vi "twoMPU.vi"() -> ()   [LabVIEW 2016]
uses:
  <vilib>/MakerHub/LINX/Private/Type Defs/Interface.ctl
  <vilib>/MakerHub/LINX/Public/Sensors/Accelerometer/MPU60X0/Clock Source.ctl
  Control 1.ctl
  <vilib>/MakerHub/LINX/Private/Type Defs/User Platform.ctl
  <vilib>/MakerHub/LINX/Public/Sensors/Accelerometer/MPU60X0/DeviceAddresses.ctl
  <vilib>/MakerHub/LINX/Public/Sensors/Accelerometer/MPU60X0/AccelFullScaleRanges.ctl
  <vilib>/MakerHub/LINX/Public/Sensors/Accelerometer/MPU60X0/GyroFullScaleRanges.ctl
  <vilib>/MakerHub/LINX/Public/Initialize.vi
  <vilib>/MakerHub/LINX/LMH-LINX.lvlib
  <vilib>/MakerHub/LINX/Public/Sensors/Accelerometer/MPU60X0/MPU60X0.lvlib
  <vilib>/Platform/NI_3dgraph.lvlib
panel:
  in  "DATA RECORD":bool
  out "XY Graph 2":cluster{"Y":dbl[], "Y":dbl[]}[](graph)
  out "Path Length 2":dbl
  in  "Baud Rate Override":T1
  in  "Clock Source 2":T2
  out "Path Length":dbl
  out "vector error":errorcluster
  in  "Plot of roll and pitch":refnum<k7>(container)
  out "XY Graph":cluster{"Y":dbl[], "Y":dbl[]}[](graph)
  out "error out":errorcluster
  out "MATLAB Error":errorcluster
  out "Error Out":errorcluster
  in  "?":bool
  in  "I2C Channel":u8
  in  "Clock Source":T2
  in  "Interface":T3
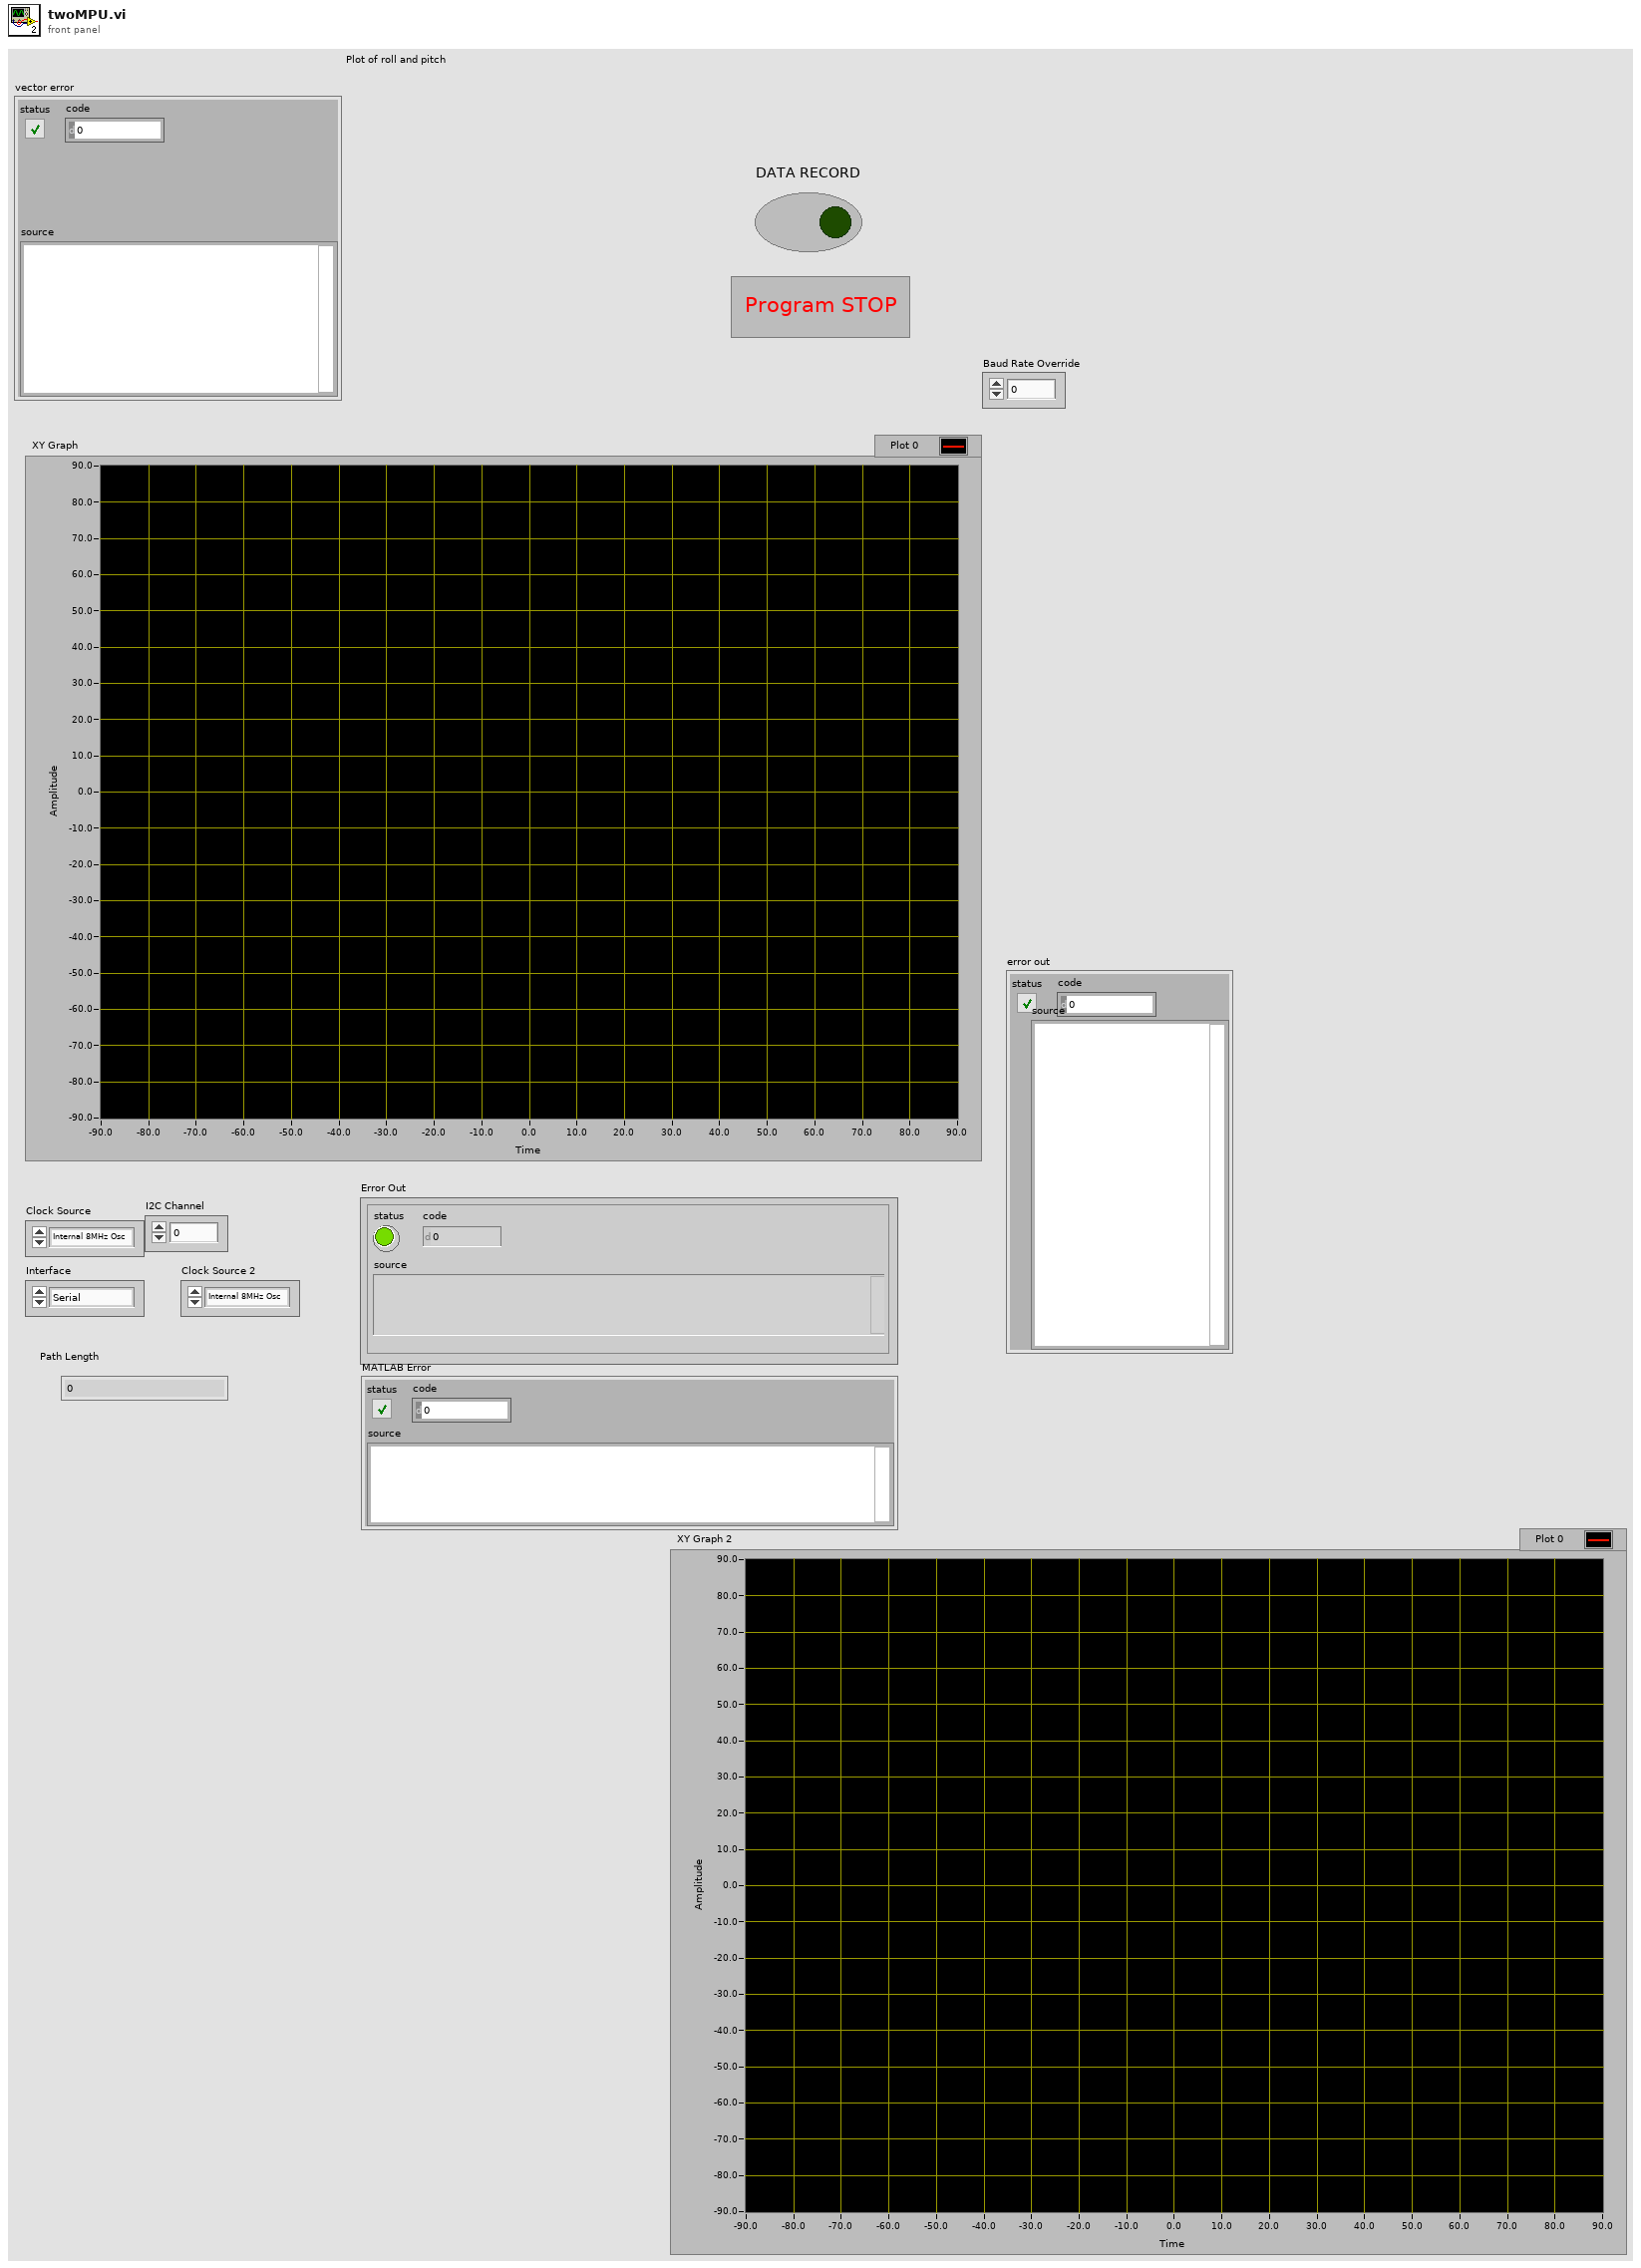
[diagram p1: front panel]
types:
  T1 = typedef "Control 1.ctl" = u32
  T2 = typedef "LMH-LINX.lvlib/MPU60X0.lvlib/Clock Source.ctl" = enum8{"Internal 8MHz Osc", "PLL with X Gyro Ref", "PLL with Y Gyro Ref", "PLL with Z Gyro Ref", "PLL with ext 32.768 KHz Ref", "PLL with ext 19.2 MHz Ref", "Reserved", "Hold in reset"}
  T3 = typedef "LMH-LINX.lvlib/Interface.ctl" = enum16{"Serial", "TCP"}
  T4 = typedef "LMH-LINX.lvlib/MPU60X0.lvlib/DeviceAddresses.ctl" = enum16{"0x68", "0x69"}
  T5 = typedef "LMH-LINX.lvlib/MPU60X0.lvlib/GyroFullScaleRanges.ctl" = enum8{"±250 °/s", "±500 °/s", "±1000 °/s", "±2000 °/s"}
  T6 = typedef "LMH-LINX.lvlib/MPU60X0.lvlib/AccelFullScaleRanges.ctl" = enum16{"±2g", "±4g", "±8g", "±16g"}
  T7 = typedef "LMH-LINX.lvlib/User Platform.ctl" = enum16{"Default", "Remote", "Local"}
  T8 = typedef "LMH-LINX.lvlib/LINX Ref.ctl" = cluster{"IO":T9, "Interface":T3, "LINX Device Config":T10}
  T9 = typedef "LMH-LINX.lvlib/Platform.ctl" = enum16{"Remote", "Local"}
  T10 = typedef "LMH-LINX.lvlib/Device.lvlib/LINX Device Config.ctl" = cluster{"Interface":T3, "COM Port":refnum<visa-resource-name>, "TCP Configuration":T11, "Device Family":u8, "Device ID":u8, "Device Name":string, "TCP Ref":refnum<k5>, "Channels":T12}
  T11 = typedef "LMH-LINX.lvlib/Device.lvlib/TCP Config.ctl" = cluster{"IP Address":string, "Port":u16}
  T12 = typedef "LMH-LINX.lvlib/Channels.ctl" = cluster{"DI":u8[], "DO":u8[], "AI":u8[], "AO":u8[], "PWM":u8[], "QE":u8[], "UART":u8[], "I2C 2":u8[], "SPI":u8[], "CAN":u8[], "Servo":u8[], "AI Ref (V)":dbl, "AI Resolution (Bits)":u8, "AO Ref (V)":dbl, "AO Resolution (Bits)":u8}
  T13 = cluster{"X Axis":i16, "Y Axis":i16, "Z Axis":i16}
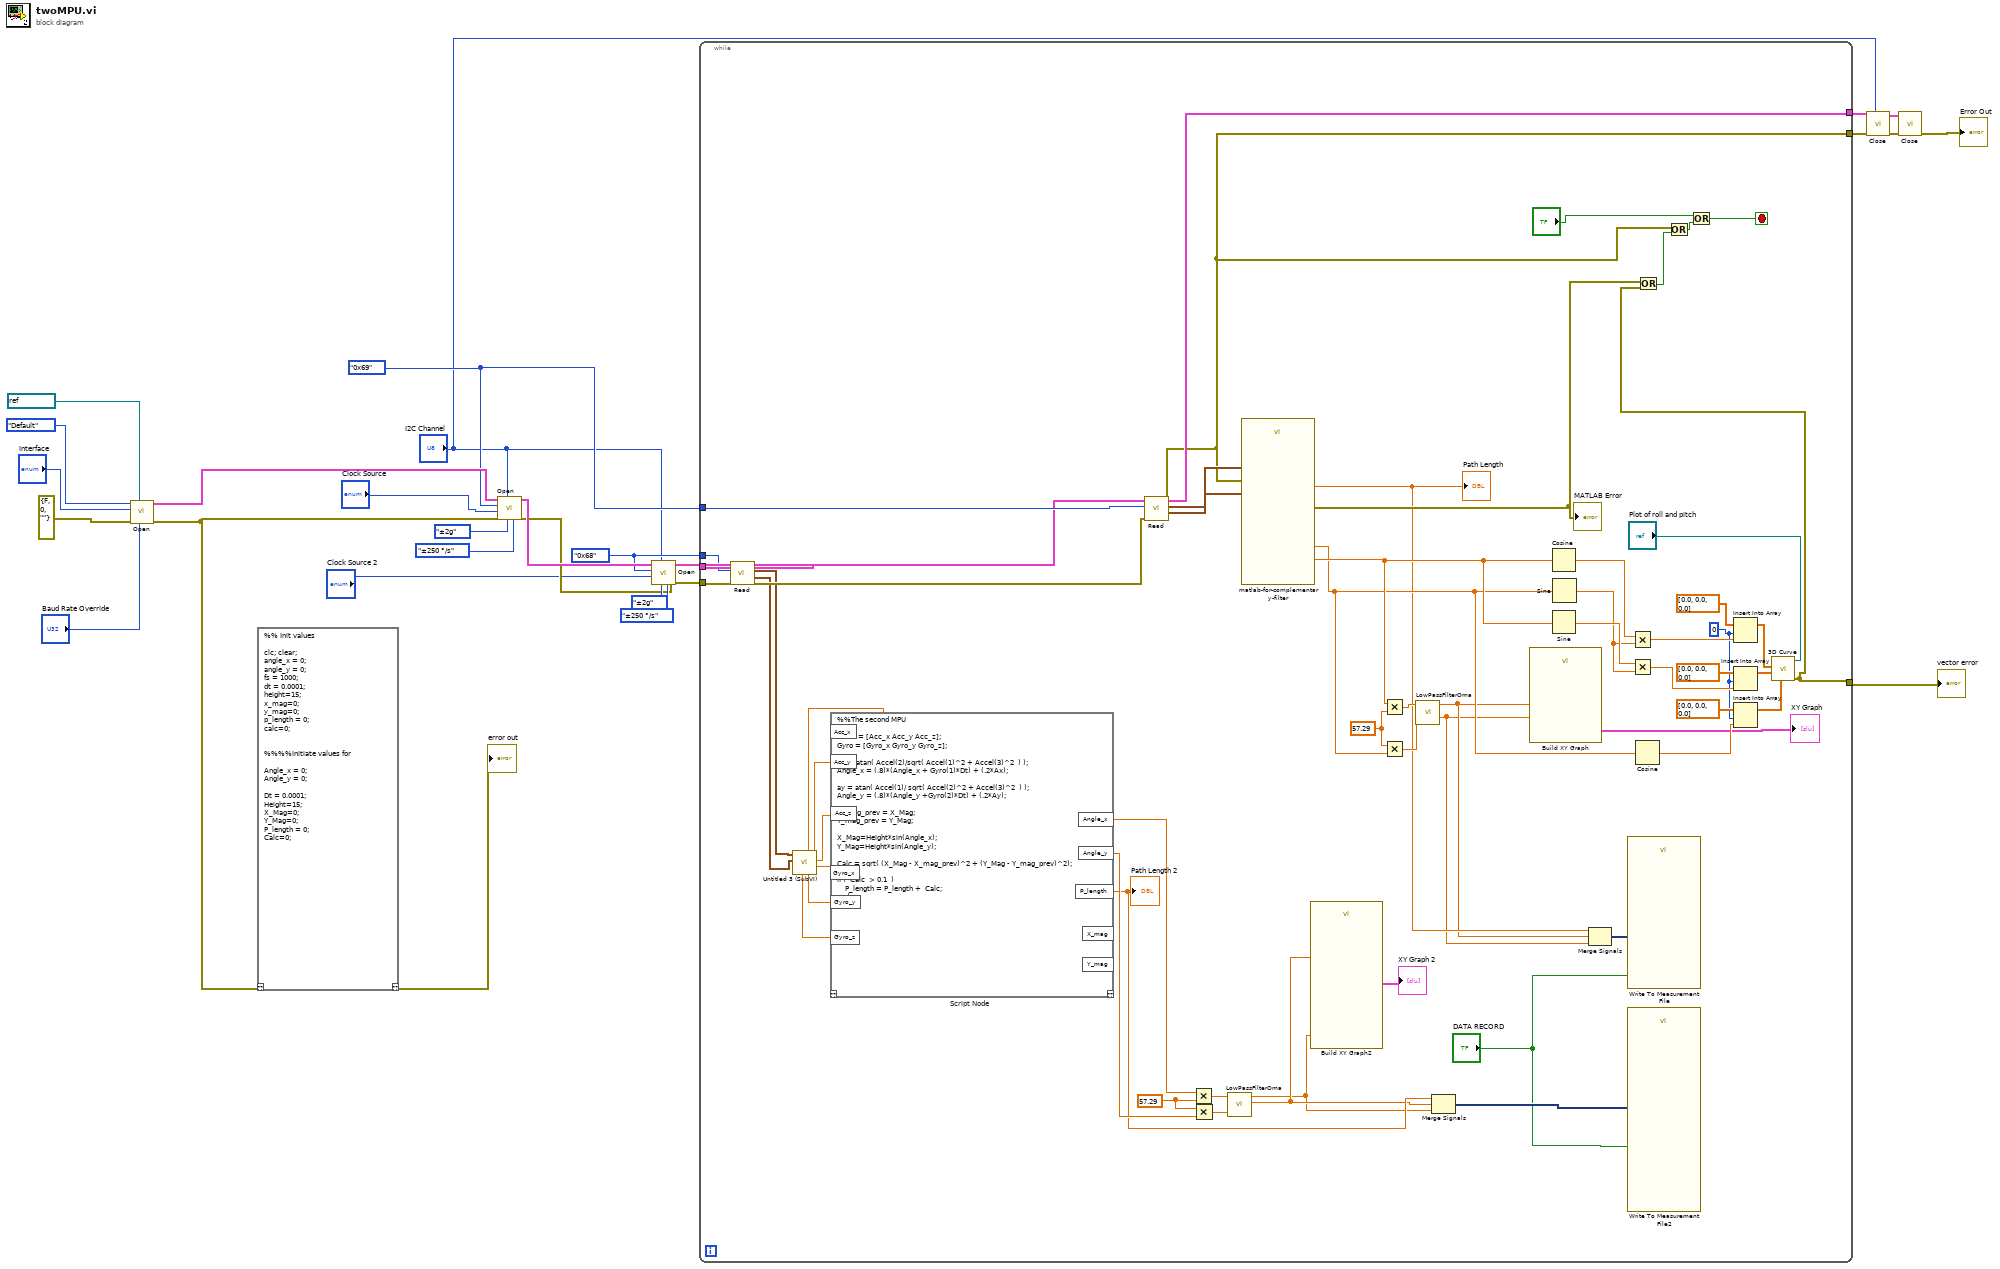
[diagram p0: block diagram]
diagram:
  w5 = DeviceAddresses."0x68" ("I2C Slave Address")
  w22 = DeviceAddresses."0x69" ("Device Address")
  n1 = call-poly <vilib>:"Open.vi"("Baud Rate Override"="Baud Rate Override", "Serial Port"=refnum<visa-resource-name> "COM3", "Error In"=errorcluster {"status"=FALSE, "code"=0, "source"=""}, "Interface"="Interface", "IO"=User_Platform."Default") -> ("Error Out"=w16:errorcluster, "LINX Resource"=w25:T8)  [unwired: 4 in, 1 out]
  n2 = script code="%% Init values\n\nclc; clear;\nangle_x = 0;\nangle_y = 0;\nfs = 1000;\ndt = 0.0001;\nheight=15;\nx_mag=0; \ny_mag=0; \np_length = 0;\ncalc=0;\n\n\n%%%%Initiate values for \n\nAngle_x = 0;\nAngle_y = 0;\n\nDt = 0.0001;\nHeight=15;\nX_Mag=0; \nY_Mag=0; \nP_length = 0;\nCalc=0;"("??"=w16) -> ("??"=→"error out":errorcluster)
  n3 = call <vilib>:"Open.vi"("Gyro Full Scale Range"=GyroFullScaleRanges."±250 °/s", "Accel Full Scale Range"=AccelFullScaleRanges."±2g", "I2C Channel"="I2C Channel", "Error In"=w16, "Clock Source"="Clock Source", "I2C Slave Address"=w22, "LINX Resource"=w25) -> ("Error Out"=w7:errorcluster, "LINX Resource"=w11:T8)  [unwired: 3 in]
  n4 = call <vilib>:"Open.vi"("Gyro Full Scale Range"=GyroFullScaleRanges."±250 °/s", "Accel Full Scale Range"=AccelFullScaleRanges."±2g", "I2C Channel"="I2C Channel", "Error In"=w7, "Clock Source"="Clock Source 2", "I2C Slave Address"=w5, "LINX Resource"=w11) -> ("Error Out"=w6:errorcluster, "LINX Resource"=w10:T8)  [unwired: 3 in]
  n5 = while {
    tunnel: w10 -> [w58]
    tunnel: w22 -> [w86]
    tunnel: [w85] -> w21
    tunnel: [w61] -> w19
    tunnel: [w62] -> w12
    tunnel: w6 -> [w55]
    tunnel: w5 -> [w56]
    stop <- w65 stop-if-true
    w36 = 57.29 ("y")
    w69 = 57.29 ("y")
    w71 = 0 ("index")
    n6 = call <vilib>:"Read.vi"("Error In"=w55, "I2C Slave Address"=w56, "LINX Resource"=w58) -> ("Error Out"=w54:errorcluster, "Gyro  Data (dps)"=w46:T13, "Acceleration Data (g)"=w47:T13, "LINX Resource"=w57:T8)  [unwired: 4 in, 1 out]
    n7 = call "Untitled 3 (SubVI).vi"("Gyro  Data (dps)"=w46, "Acceleration Data (g)"=w47) -> ("Gyro_X"=w42:dbl, "Accel_Z"=w43:dbl, "Accel_Y"=w44:dbl, "Gyro_Y"=w41:dbl, "Accel_X"=w45:dbl, "Gyro_Z"=w40:dbl)  [unwired: 4 in]
    n8 = script code="%%The second MPU \n\nAccel = [Acc_x Acc_y Acc_z];\nGyro = [Gyro_x Gyro_y Gyro_z];\n\nAx = atan( Accel(2)/sqrt( Accel(1)^2 + Accel(3)^2  ) );\nAngle_x = (.8)*(Angle_x + Gyro(1)*Dt) + (.2*Ax);\n\nay = atan( Accel(1)/ sqrt( Accel(2)^2 + Accel(3)^2  ) );\nAngle_y = (.8)*(Angle_y +Gyro(2)*Dt) + (.2*Ay);\n\nX_mag_prev = X_Mag;\nY_mag_prev = Y_Mag;\n\nX_Mag=Height*sin(Angle_x); \nY_Mag=Height*sin(Angle_y);\n\nCalc = sqrt( (X_Mag - X_mag_prev)^2 + (Y_Mag - Y_mag_prev)^2);\n\nif (  Calc  > 0.1  ) \n    P_length = P_length +  Calc;\nend" "Script Node"("Acc_x"=w45, "Acc_y"=w44, "Acc_z"=w43, "Gyro_x"=w42, "Gyro_y"=w41, "Gyro_z"=w40) -> ("Angle_x"=w35:dbl, "Angle_y"=w34:dbl, "P_length"=w31:dbl)  [unwired: 1 in, 3 out]
    "Path Length 2" <- w31
    n9 = call <vilib>:"Read.vi"("Error In"=w54, "I2C Slave Address"=w86, "LINX Resource"=w57) -> ("Error Out"=w61:errorcluster, "Gyro  Data (dps)"=w83:T13, "Acceleration Data (g)"=w84:T13, "LINX Resource"=w85:T8)  [unwired: 4 in, 1 out]
    n10 = Multiply(x=w35, y=w36) -> (x*y=w38:dbl)
    n11 = Multiply(x=w36, y=w34) -> (x*y=w37:dbl)
    n12 = call "LowPassFilterOma.vi"("Numeric"=w37, "Numeric 2"=w38) -> ("Filtered x"=w30:dbl, "Filtered x 2"=w29:dbl)  [unwired: 8 in]
    n13 = call "matlab-for-complementary-filter.vi"("Acceleration Data (g)"=w84, "Gyro  Data (dps)"=w83, "error in (no error)"=w61) -> ("angle_y"=w70:dbl, "Path Length"=w50:dbl, "angle_x"=w68:dbl, "error out"=w63:errorcluster)  [unwired: 11 in, 2 out]
    "MATLAB Error" <- w63
    "Path Length" <- w50
    n14 = call "Build XY Graph2"("Y Input"=w29, "X Input"=w30) -> ("XY Graph"=→"XY Graph 2":cluster{"X":dbl[], "Y":dbl[]}[])  [unwired: 8 in, 1 out]
    n15 = Multiply(x=w70, y=w69) -> (x*y=w53:dbl)
    n16 = Multiply(x=w69, y=w68) -> (x*y=w52:dbl)
    n17 = call "LowPassFilterOma.vi"("Numeric"=w52, "Numeric 2"=w53) -> ("Filtered x"=w48:dbl, "Filtered x 2"=w49:dbl)  [unwired: 8 in]
    n18 = Merge Signals(w31, w30, w29) -> (w39:dynamicdata)
    n19 = call "Build XY Graph"("Y Input"=w48, "X Input"=w49) -> ("XY Graph"=→"XY Graph":cluster{"X":dbl[], "Y":dbl[]}[])  [unwired: 8 in, 1 out]
    n20 = Cosine(x=w70) -> (cos(x)=w82:dbl)
    n21 = Sine(x=w70) -> (sin(x)=w77:dbl)
    n22 = Sine(x=w68) -> (sin(x)=w76:dbl)
    n23 = Merge Signals(w50, w49, w48) -> (w51:dynamicdata)
    n24 = call "Write To Measurement File"("Signals"=w51, "Enable"="DATA RECORD") -> ()  [unwired: 15 in, 3 out]
    n25 = call "Write To Measurement File2"("Signals"=w39, "Enable"="DATA RECORD") -> ()  [unwired: 15 in, 3 out]
    n26 = Multiply(x=w82, y=w76) -> (x*y=w79:dbl)
    n27 = Multiply(x=w77, y=w76) -> (x*y=w75:dbl)
    n28 = Cosine(x=w68) -> (cos(x)=w73:dbl)
    n29 = Insert Into Array(array=dbl[] [0.0, 0.0, 0.0], index=w71, new element=w79) -> (w67:dbl[])
    n30 = Insert Into Array(array=dbl[] [0.0, 0.0, 0.0], index=w71, new element=w75) -> (w66:dbl[])
    n31 = Insert Into Array(array=dbl[] [0.0, 0.0, 0.0], index=w71, new element=w73) -> (w72:dbl[])
    n32 = call <vilib>:"3D Curve.vi"("z vector"=w72, "y vector"=w66, "x vector"=w67, "3D graph"="Plot of roll and pitch") -> ("error out"=w62:errorcluster)  [unwired: 6 in, 1 out]
    n33 = Or(x=w63, y=w62) -> (x .or. y?=w64:bool)
    n34 = Or(x=w61, y=w64) -> (x .or. y?=w59:bool)
    n35 = Or(x="?", y=w59) -> (x .or. y?=w65:bool)
  }
  "vector error" <- w12
  n36 = call <vilib>:"Close.vi"("I2C Channel (0)"="I2C Channel", "Error In"=w19, "LINX Resource"=w21) -> ("Error Out"=w18:errorcluster, "LINX Resource"=w20:T8)  [unwired: 7 in]
  n37 = call <vilib>:"Close.vi"("Error In"=w18, "LINX Resource"=w20) -> ("Error Out"=→"Error Out":errorcluster)  [unwired: 9 in]
